vi "Get Transfer Group Parameters.vi"(11 "GE Reflective Memory in":refnum<class "GE Reflective Memory Transceiver.lvclass">) -> (2 "Transfer Group Parameters":T1[](array[typedef]) {"DMA Transfer Specs"."Block Descriptors"."descriptor params"."data ptr (lower)" format="%.0x"; "DMA Transfer Specs"."Block Descriptors"."descriptor params"."data ptr (upper)" format="%.0x"; "DMA Transfer Specs"."Block Descriptors"."descriptor params"."data size" format="%.0x"; "DMA Transfer Specs"."Block Descriptors"."descriptor params"."next descriptor ptr" format="%.0x"; "DMA Transfer Specs"."Block Descriptors"."descriptor size" format="%08x"; "DMA Transfer Specs"."Block Descriptors"."descriptor ptr (RFM)" format="%08x"; "DMA Transfer Specs"."Block Descriptors"."descriptor ptr (VISA)" format="%08x"; "DMA Transfer Specs"."RFM offset" format="%08x"}, 3 "GE Reflective Memory out":refnum<class "GE Reflective Memory Transceiver.lvclass">)   [LabVIEW 2020, in "GE Reflective Memory.lvlib" / "GE Reflective Memory Transceiver.lvclass"]
uses:
  GE Reflective Memory Transceiver.lvclass
  Transfer Group Parameters.ctl
  Driver/Source/Typedefs/GE 5565PIORC.Typedef.DMA Transfer Spec.ctl
  Driver/Source/Typedefs/GE 5565PIORC.Typedef.DMA Block Descriptor.ctl
  Driver/Source/Typedefs/GE 5565PIORC.Typedef.DMA Block Descriptor Params.ctl
  GE Reflective Memory Transceiver.lvclass/GE Reflective Memory Transceiver.ctl
  Driver/Source/GE 5565PIORC.lvclass
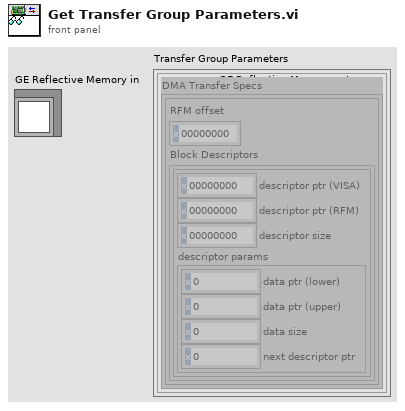
[diagram p1: front panel]
types:
  T1 = typedef "GE Reflective Memory.lvlib/GE Reflective Memory Transceiver.lvclass/Transfer Group Parameters.ctl" = cluster{"DMA Transfer Specs":T2[]}
  T2 = typedef "GE 5565PIORC.lvclass/GE 5565PIORC.Typedef.DMA Transfer Spec.ctl" = cluster{"RFM offset":u32, "Block Descriptors":T3[]}
  T3 = typedef "GE 5565PIORC.lvclass/GE 5565PIORC.Typedef.DMA Block Descriptor.ctl" = cluster{"descriptor ptr (VISA)":u32, "descriptor ptr (RFM)":u32, "descriptor size":u32, "descriptor params":T4}
  T4 = typedef "GE 5565PIORC.lvclass/GE 5565PIORC.Typedef.DMA Block Descriptor Params.ctl" = cluster{"data ptr (lower)":u32, "data ptr (upper)":u32, "data size":u32, "next descriptor ptr":u32}
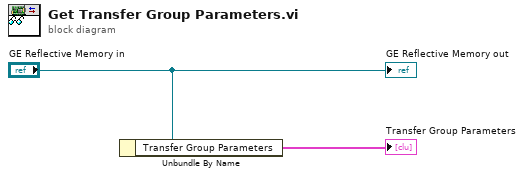
[diagram p0: block diagram]
diagram:
  n1 = Unbundle By Name("GE Reflective Memory in") -> ("Transfer Group Parameters"=→"Transfer Group Parameters":T1[])
  "GE Reflective Memory out" <- "GE Reflective Memory in"
